vi "Sweep single SMU.vi"() -> ()   [LabVIEW 2018]
uses:
  C/Program Files/National Instruments/LabVIEW 2021/instr.lib/Keithley 2450/Keithley 2450.lvlib
  C/Program Files/National Instruments/LabVIEW 2021/instr.lib/Keithley 2450/Public/Data/Read (Multiple Points).vi
panel:
  in  "Delay (0) in Sec":dbl=0.001 format="%#_13g"
  in  "Measurement Speed (1 PLC)":dbl=1.0 format="%#_13g"
  in  "Limit  Level (0.1)":dbl=0.1 format="%#_13g"
  out "Waveform Graph":dbl[][](graph)
  in  "VISA resource name":refnum<visa-resource-name>
  in  "Sweep Points":T1={"Start "=1.0, "Stop "=0.0, "Number of Points (5)"=5}
  in  "Source Mode  (0: Voltage)":u16(ring) items=["Voltage", "Current"]
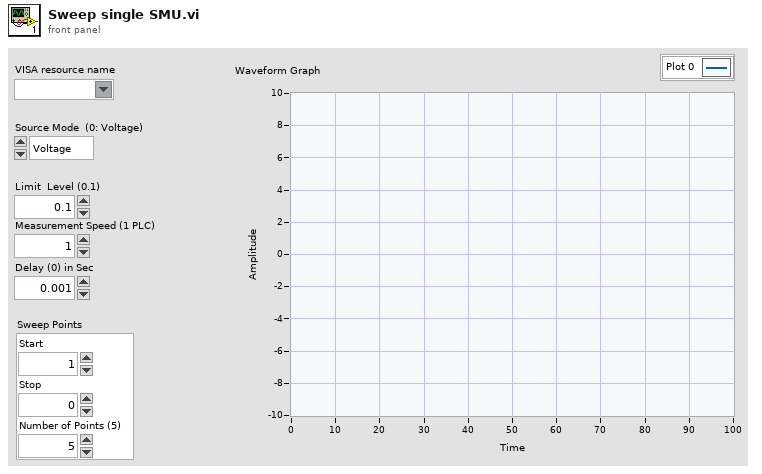
[diagram p1: front panel]
types:
  T1 = cluster{"Start ":dbl, "Stop ":dbl, "Number of Points (5)":u32}
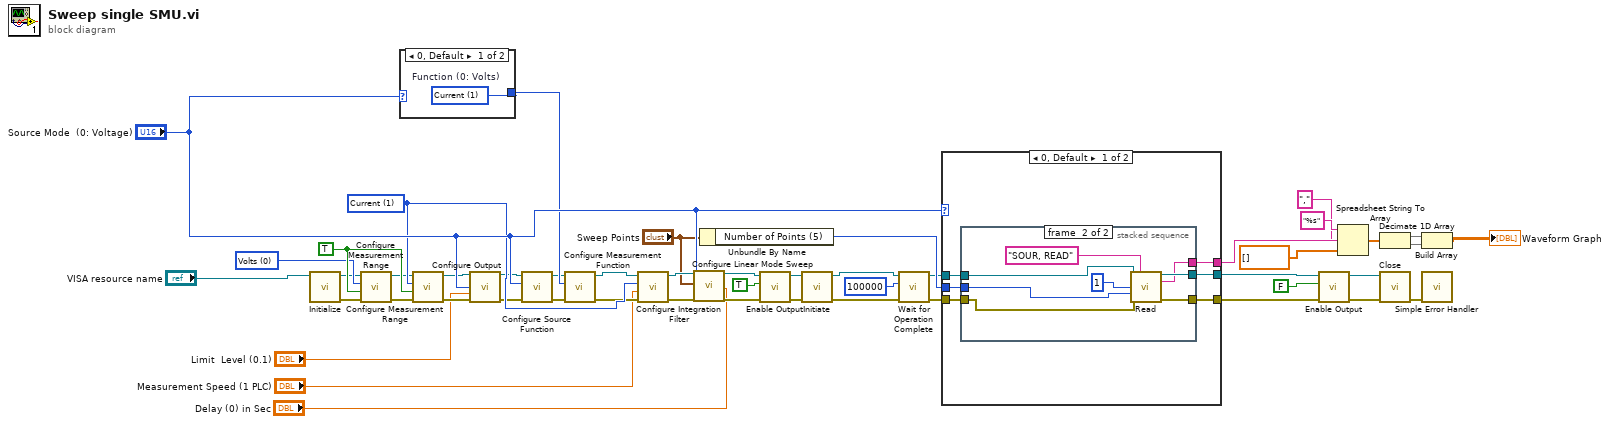
[diagram p0: block diagram]
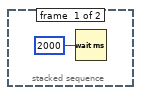
[diagram p2: hidden frame]
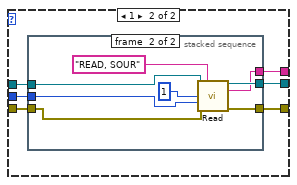
[diagram p3: hidden frame]
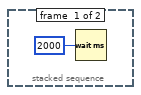
[diagram p4: hidden frame]
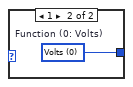
[diagram p5: hidden frame]
diagram:
  w41 = u16 1 items=["Volts", "Current", "Resistance"] ("Function (0: Volts) 2")
  w12 = u16 0 items=["Volts", "Current", "Resistance"] ("Function (0: Volts)")
  w13 = TRUE ("Enable Auto Range (T:Enable)")
  n1 = call "Initialize.vi"("VISA resource name"="VISA resource name") -> ("error out"=w4:errorcluster, "VISA resource name out"=w3:refnum<visa-resource-name>)  [unwired: 9 in]
  n2 = call "Configure Measurement Range.vi"("error in (no error)"=w4, "Enable Auto Range (T:Enable)"=w13, "Function (0: Volts)"=w12, "VISA resource name"=w3) -> ("error out"=w5:errorcluster, "VISA resource name out"=w6:refnum<visa-resource-name>)  [unwired: 6 in]
  n3 = case shown="0, Default" "Source Mode  (0: Voltage)" {
    tunnel: [w50 w51] -> w42
    frame 0, Default {
      w50 = u16 1 items=["Volts", "Current", "Resistance"]  # Function (0: Volts)
    }
    frame 1 {
      w51 = u16 0 items=["Volts", "Current", "Resistance"]  # Function (0: Volts)
    }
  }
  n4 = call "Configure Measurement Range.vi"("error in (no error)"=w5, "Enable Auto Range (T:Enable)"=w13, "Function (0: Volts)"=w41, "VISA resource name"=w6) -> ("error out"=w16:errorcluster, "VISA resource name out"=w15:refnum<visa-resource-name>)  [unwired: 6 in]
  n5 = call "Configure Output.vi"("VISA resource name"=w15, "Source Mode  (0: Voltage)"="Source Mode  (0: Voltage)", "Source Limit Level (0.1)"="Limit  Level (0.1)", "error in (no error)"=w16) -> ("VISA resource name out"=w18:refnum<visa-resource-name>, "error out"=w17:errorcluster)  [unwired: 10 in]
  n6 = call "Configure Source Function.vi"("error in (no error)"=w17, "Function (0: Volts)"="Source Mode  (0: Voltage)", "VISA resource name"=w18) -> ("error out"=w38:errorcluster, "VISA resource name out"=w37:refnum<visa-resource-name>)  [unwired: 7 in]
  n7 = call "Configure Measurement Function.vi"("error in (no error)"=w38, "Function (0: Volts)"=w42, "VISA resource name"=w37) -> ("error out"=w39:errorcluster, "VISA resource name out"=w40:refnum<visa-resource-name>)  [unwired: 7 in]
  n8 = call "Configure Integration Filter.vi"("error in (no error)"=w39, "Measurement Speed (1 PLC)"="Measurement Speed (1 PLC)", "Function (0: Volts)"=w41, "VISA resource name"=w40) -> ("error out"=w33:errorcluster, "VISA resource name out"=w34:refnum<visa-resource-name>)  [unwired: 6 in]
  n9 = call "Configure Linear Mode Sweep.vi"("VISA resource name"=w34, "Source Mode  (0: Voltage)"="Source Mode  (0: Voltage)", "Sweep Points"="Sweep Points", "Delay (0)"="Delay (0) in Sec", "error in (no error)"=w33) -> ("VISA resource name out"=w20:refnum<visa-resource-name>, "error out"=w21:errorcluster)  [unwired: 13 in]
  n10 = Unbundle By Name("Sweep Points") -> ("Number of Points (5)"=w48:u32)
  n11 = call "Enable Output.vi"("error in (no error)"=w21, "Enable Output (T: Enable)"=TRUE, "VISA resource name"=w20) -> ("error out"=w23:errorcluster, "VISA resource name out"=w22:refnum<visa-resource-name>)  [unwired: 7 in]
  n12 = call "Initiate.vi"("error in (no error)"=w23, "VISA resource name"=w22) -> ("error out"=w32:errorcluster, "VISA resource name out"=w31:refnum<visa-resource-name>)  [unwired: 8 in]
  n13 = call "Wait for Operation Complete.vi"("error in (no error)"=w32, "Timeout (10000 ms)"=100000, "VISA resource name"=w31) -> ("error out"=w45:errorcluster, "VISA resource name out"=w44:refnum<visa-resource-name>)  [unwired: 7 in]
  n14 = case shown="0, Default" "Source Mode  (0: Voltage)" {
    tunnel: w44 -> [w57 w72]
    tunnel: w45 -> [w56 w71]
    tunnel: [w55 w69] -> w46
    tunnel: [w54 w68] -> w47
    tunnel: w48 -> [w53 w70]
    tunnel: [w52 w67] -> w49
    frame 0, Default {
      n15 = stacked-sequence {
        tunnel: [_ w66] -> w55
        tunnel: [_ w65] -> w54
        tunnel: w57 -> [_ w63]
        tunnel: w56 -> [_ w62]
        tunnel: [_ w61] -> w52
        tunnel: w53 -> [_ w59]
        frame #0 {
          n16 = Wait (ms)(milliseconds to wait=u32 2000) -> ()  [unwired: 1 out]
        }
        frame #1 {
          n17 = call-poly "Read.vi"("VISA resource name"=w63, "Buffer Elements"="SOUR, READ", "Start Index (1)"=1, "End Index (1)"=w59, "error in (no error)"=w62) -> ("VISA resource name out"=w66:refnum<visa-resource-name>, "Data out"=w61:string, "error out"=w65:errorcluster)  [unwired: 8 in]
        }
      }
    }
    frame 1 {
      n18 = stacked-sequence {
        tunnel: [_ w81] -> w69
        tunnel: [_ w80] -> w68
        tunnel: w72 -> [_ w78]
        tunnel: w71 -> [_ w77]
        tunnel: [_ w76] -> w67
        tunnel: w70 -> [_ w74]
        frame #0 {
          n19 = Wait (ms)(milliseconds to wait=u32 2000) -> ()  [unwired: 1 out]
        }
        frame #1 {
          n20 = call-poly "Read.vi"("VISA resource name"=w78, "Buffer Elements"="READ, SOUR", "Start Index (1)"=1, "End Index (1)"=w74, "error in (no error)"=w77) -> ("VISA resource name out"=w81:refnum<visa-resource-name>, "Data out"=w76:string, "error out"=w80:errorcluster)  [unwired: 8 in]
        }
      }
    }
  }
  n21 = call "Enable Output.vi"("error in (no error)"=w47, "Enable Output (T: Enable)"=FALSE, "VISA resource name"=w46) -> ("error out"=w9:errorcluster, "VISA resource name out"=w8:refnum<visa-resource-name>)  [unwired: 7 in]
  n22 = Spreadsheet String To Array(delimiter (Tab)=",", format string="%s", spreadsheet string=w49, array type (2D Dbl)=dbl[] []) -> (array=w28:dbl[])
  n23 = Decimate 1D Array(w28) -> (w29:dbl[], w30:dbl[])
  n24 = call "Close.vi"("error in (no error)"=w9, "VISA resource name"=w8) -> ("error out"=w7:errorcluster)  [unwired: 9 in]
  n25 = Build Array(w29, w30) -> (→"Waveform Graph":dbl[][])
  n26 = call <vilib>:"Simple Error Handler.vi"("error in (no error)"=w7) -> ()  [unwired: 4 in, 5 out]
